vi "PH_SSAC.PC Global On.vi"(0 "i ref in":refnum<vi>, 2 "Global On?":bool, 5 "error in (no error)":errorcluster) -> (14 "i ref out":refnum<vi>, 19 "error out":errorcluster)   [LabVIEW 2014, in "PH_SSAC.lvlib"]
doc: "This is the Proc Case \"Remote Control\"."
uses:
  PH_SSAC.lvlib
  PH_Common/PH_Common.lvlib
  CSCore/BaseProcess/BaseProcess.lvlib
  PH_Img_BaseClass/PH_Img_BaseClass.lvlib
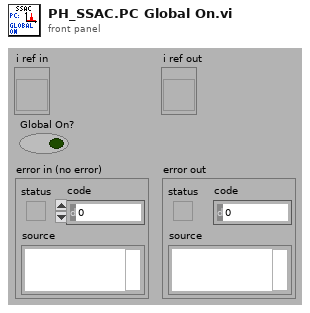
[diagram p1: front panel]
types:
  T1 = typedef "PH_Img_BaseClass.lvlib/PH_Img_BaseClass.i attribute.ctl" = cluster{"GUI Refs":T2, "Timeout Image [ms]":i32, "Default Periodic Period [ms]":i32, "Camera":cluster{"Instancename":string, "Notifier":refnum<notifier>}, "Palette":T3, "Cam Settings":cluster{"Cam ID":string, "Gain":dbl, "Brightness":dbl, "Shutter":dbl, "Cam Info Failure":bool, "Mode":i32}}
  T2 = typedef "PH_Img_BaseClass.lvlib/PH_Img_BaseClass.GUI Refs.ctl" = cluster{"Timeout":refnum<vi>, "Image":refnum<vi>, "Palette":refnum<vi>, "Timeout Set":refnum<vi>}
  T3 = typedef "PH_Img_BaseClass.lvlib/PH_Img_BaseClass.Palette.ctl" = i32
  T4 = typedef "PH_SSAC.lvlib/PH_SSAC.i attribute.ctl" = cluster{"GUI Refs":cluster{"Delete":refnum<vi>, "Global On":refnum<vi>, "Cam Source":refnum<vi>, "Frame Main Signal":refnum<vi>, "Frame Background":refnum<vi>, "dt (Gauss smooth)":refnum<vi>, "Calibration Factor":refnum<vi>, "Background acquire":refnum<vi>, "Threshold":refnum<vi>, "Time evolution of mean pulse duration":refnum<vi>, "Mean Pulse Duration":refnum<vi>, "Main signal":refnum<vi>, "Current Pulse Duration":refnum<vi>, "Processed":refnum<vi>, "Saturation":refnum<vi>, "# for Average":refnum<vi>, "Position":refnum<vi>, "BG Status":refnum<vi>, "Save BG data":refnum<vi>, "Read BG Data":refnum<vi>, "Background Calibration Data":refnum<vi>}, "Images":cluster{"OP Image":T5, "GUI Image":T5, "PSDB Image":T5}, "Global On?":bool, "Frame Main":cluster{"x":u32, "dx":u32, "y":u32, "dy":u32}, "Frame Background":cluster{"x":u32, "dx":u32, "y":u32, "dy":u32}, "dt [fs]":dbl, "Calibration Factor [fs/pixel]":dbl, "Threshold":dbl, "Time evolution of mean pulse duration [fs]":dbl[], "Main Signal":cluster{"Time for Main":dbl[], "Signal":dbl[]}, "Processed":bool, "Current Pulse Duration [fs]":dbl, "# for Average":i32, "Position":i32, "Pulse Durations [fs]":dbl[], "BG":cluster{"Acquire?":bool, "Background Calibration Data":T6, "Save Data":bool}}
  T5 = typedef "IMAQ Image.ctl" = refnum<image>
  T6 = typedef "PH_SSAC.lvlib/PH_SSAC.Background Data.ctl" = cluster{"Date":string, "Time":string, "Frame Main":cluster{"x":u32, "dx":u32, "y":u32, "dy":u32}, "dt [fs]":dbl, "Calibration Factor [fs/pixel]":dbl, "Signal":dbl[], "Frame Background":cluster{"x":u32, "dx":u32, "y":u32, "dy":u32}}
  T7 = enum16{"simple", "synchronous", "asynchronous", "notification"}
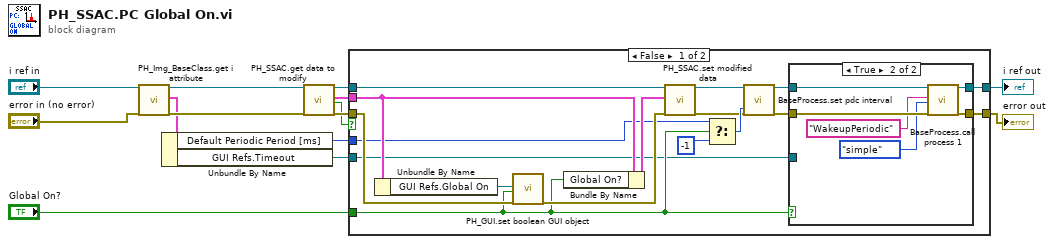
[diagram p0: block diagram]
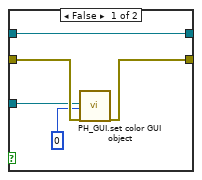
[diagram p2: hidden frame]
diagram:
  n1 = call "PH_Img_BaseClass.get i attribute.vi"("i ref in"="i ref in", "error in (no error)"="error in (no error)") -> ("i ref out"=w6:refnum<vi>, "i attribute"=w3:T1, "error out"=w4:errorcluster)  [unwired: 15 in]
  n2 = Unbundle By Name(w3) -> ("Default Periodic Period [ms]"=w1:i32, "GUI Refs.Timeout"=w2:refnum<vi>)
  n3 = call "PH_SSAC.get data to modify.vi"("i ref in"=w6, "error in (no error)"=w4) -> ("i ref out"=w13:refnum<vi>, "i attribute"=w10:T4, "timed out"=w8:bool, "error out"=w14:errorcluster)  [unwired: 14 in]
  n4 = case shown="False" w8 {
    tunnel: w14 -> [w31 w43]
    tunnel: w13 -> [w30 w44]
    tunnel: [w26 w44] -> w12
    tunnel: [w24 w43] -> w11
    tunnel: w10 -> [w20 _]
    tunnel: "Global On?" -> [w18 _]
    tunnel: w2 -> [w16 _]
    tunnel: w1 -> [w15 _]
    frame False {
      n5 = Unbundle By Name(w20) -> ("GUI Refs.Global On"=w17:refnum<vi>)
      n6 = call "PH_GUI.set boolean GUI object.vi"("Boolean Knob GUI Ref"=w17, "Value"=w18, "error in (no error)"=w31) -> ("error out"=w22:errorcluster)  [unwired: 16 in]
      n7 = Bundle By Name(cluster=w20, "Global On?"=w18) -> (w19:T4)
      n8 = call "PH_SSAC.set modified data.vi"("i ref in"=w30, "i attribute"=w19, "error in (no error)"=w22) -> ("i ref out"=w23:refnum<vi>, "error out"=w21:errorcluster)  [unwired: 15 in]
      n9 = Select(t=w15, s=w18, f=-1) -> (s? t:f=w28:i32)
      n10 = call "BaseProcess.set pdc interval.vi"("i ref in"=w23, "PeriodicInterval [ms]"=w28, "error in (no error)"=w21) -> ("i ref out"=w27:refnum<vi>, "error out"=w25:errorcluster)  [unwired: 14 in, 1 out]
      n11 = case shown="True" w18 {
        tunnel: [w32 w42] -> w26
        tunnel: w25 -> [w35 w41]
        tunnel: [w36 w40] -> w24
        tunnel: w27 -> [w32 w39]
        tunnel: w16 -> [w34 _]
        frame False {
          n12 = call "PH_GUI.set color GUI object.vi"("GUI object Ref"=w34, "State"=0, "error in (no error)"=w35) -> ("error out"=w36:errorcluster)  [unwired: 16 in]
        }
        frame True {
          n13 = call "BaseProcess.call process 1.vi"("i ref in"=w39, "Selector"="WakeupPeriodic", "CallType"=T7."simple", "error in (no error)"=w41) -> ("i ref out"=w42:refnum<vi>, "error out"=w40:errorcluster)  [unwired: 13 in, 1 out]
        }
      }
    }
    frame True {
    }
  }
  "i ref out" <- w12
  "error out" <- w11
